vi "Funnel_global.vi"() -> ()   [LabVIEW 2020]
uses:
  Subsystems/Funnel/Funnel_Cluster.ctl
  Subsystems/Funnel/Control_States_Funnel.ctl
panel:
  in  "Funnel_Output":dbl
  in  "Funnel_Execute_Notifier":refnum<notifier>
  in  "Funnel_Set_Notifier":refnum<notifier>
  in  "Funnel_Set_Ref":string="Funnel_Set_Ref"
  in  "Funnel_Execute_Ref":string="Funnel_Execute_Ref"
  in  "Funnel_Motor_Ref":string="Funnel_Motor_Ref"
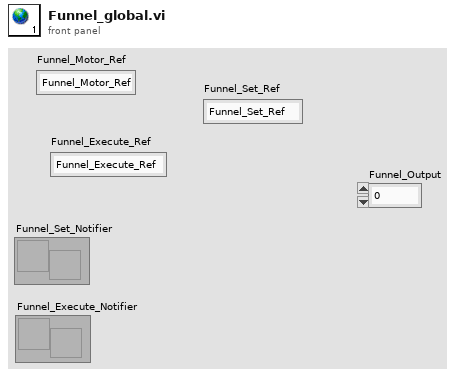
[diagram p1: front panel]
diagram:
